vi "LoadUtilization.vi"(0 "base path":path=path "c:/temp", 2 "machine":string="QAMT01") -> (7 "appended array":string[](array[string]), 9 "error out":errorcluster)   [LabVIEW 2012]
uses:
  <vilib>/addons/database/Connection.llb/DB Tools Open Connec (Path).vi
  <vilib>/Utility/file.llb/Read From Spreadsheet File (string).vi
  <vilib>/addons/database/Connection.llb/Conn Execute.vi
  <vilib>/addons/database/Recordset.llb/Rec Fetch Integer Data (R).vi
  <vilib>/addons/database/Recordset.llb/Rec Destroy - Connection.vi
  <vilib>/regexp/Match Regular Expression.xnode
  <vilib>/addons/database/NI_Database_API.lvlib
panel:
  out "error out 4":errorcluster
  out "error out 3":errorcluster
  out "input cluster 2":T1
  out "error out 2":errorcluster
  out "trimmed string":string
  out "output cluster":T1
  out "data":i32
  out "concatenated string":string
  out "x = y?":bool
  in  "input cluster":T1
  in  "String":string
  in  "Array":string[](array[string])
  out "filenames":string[](array[string])
  out "Numeric":i32
  in  "date/time string 2":string
  out "all rows":string[][](array[string])
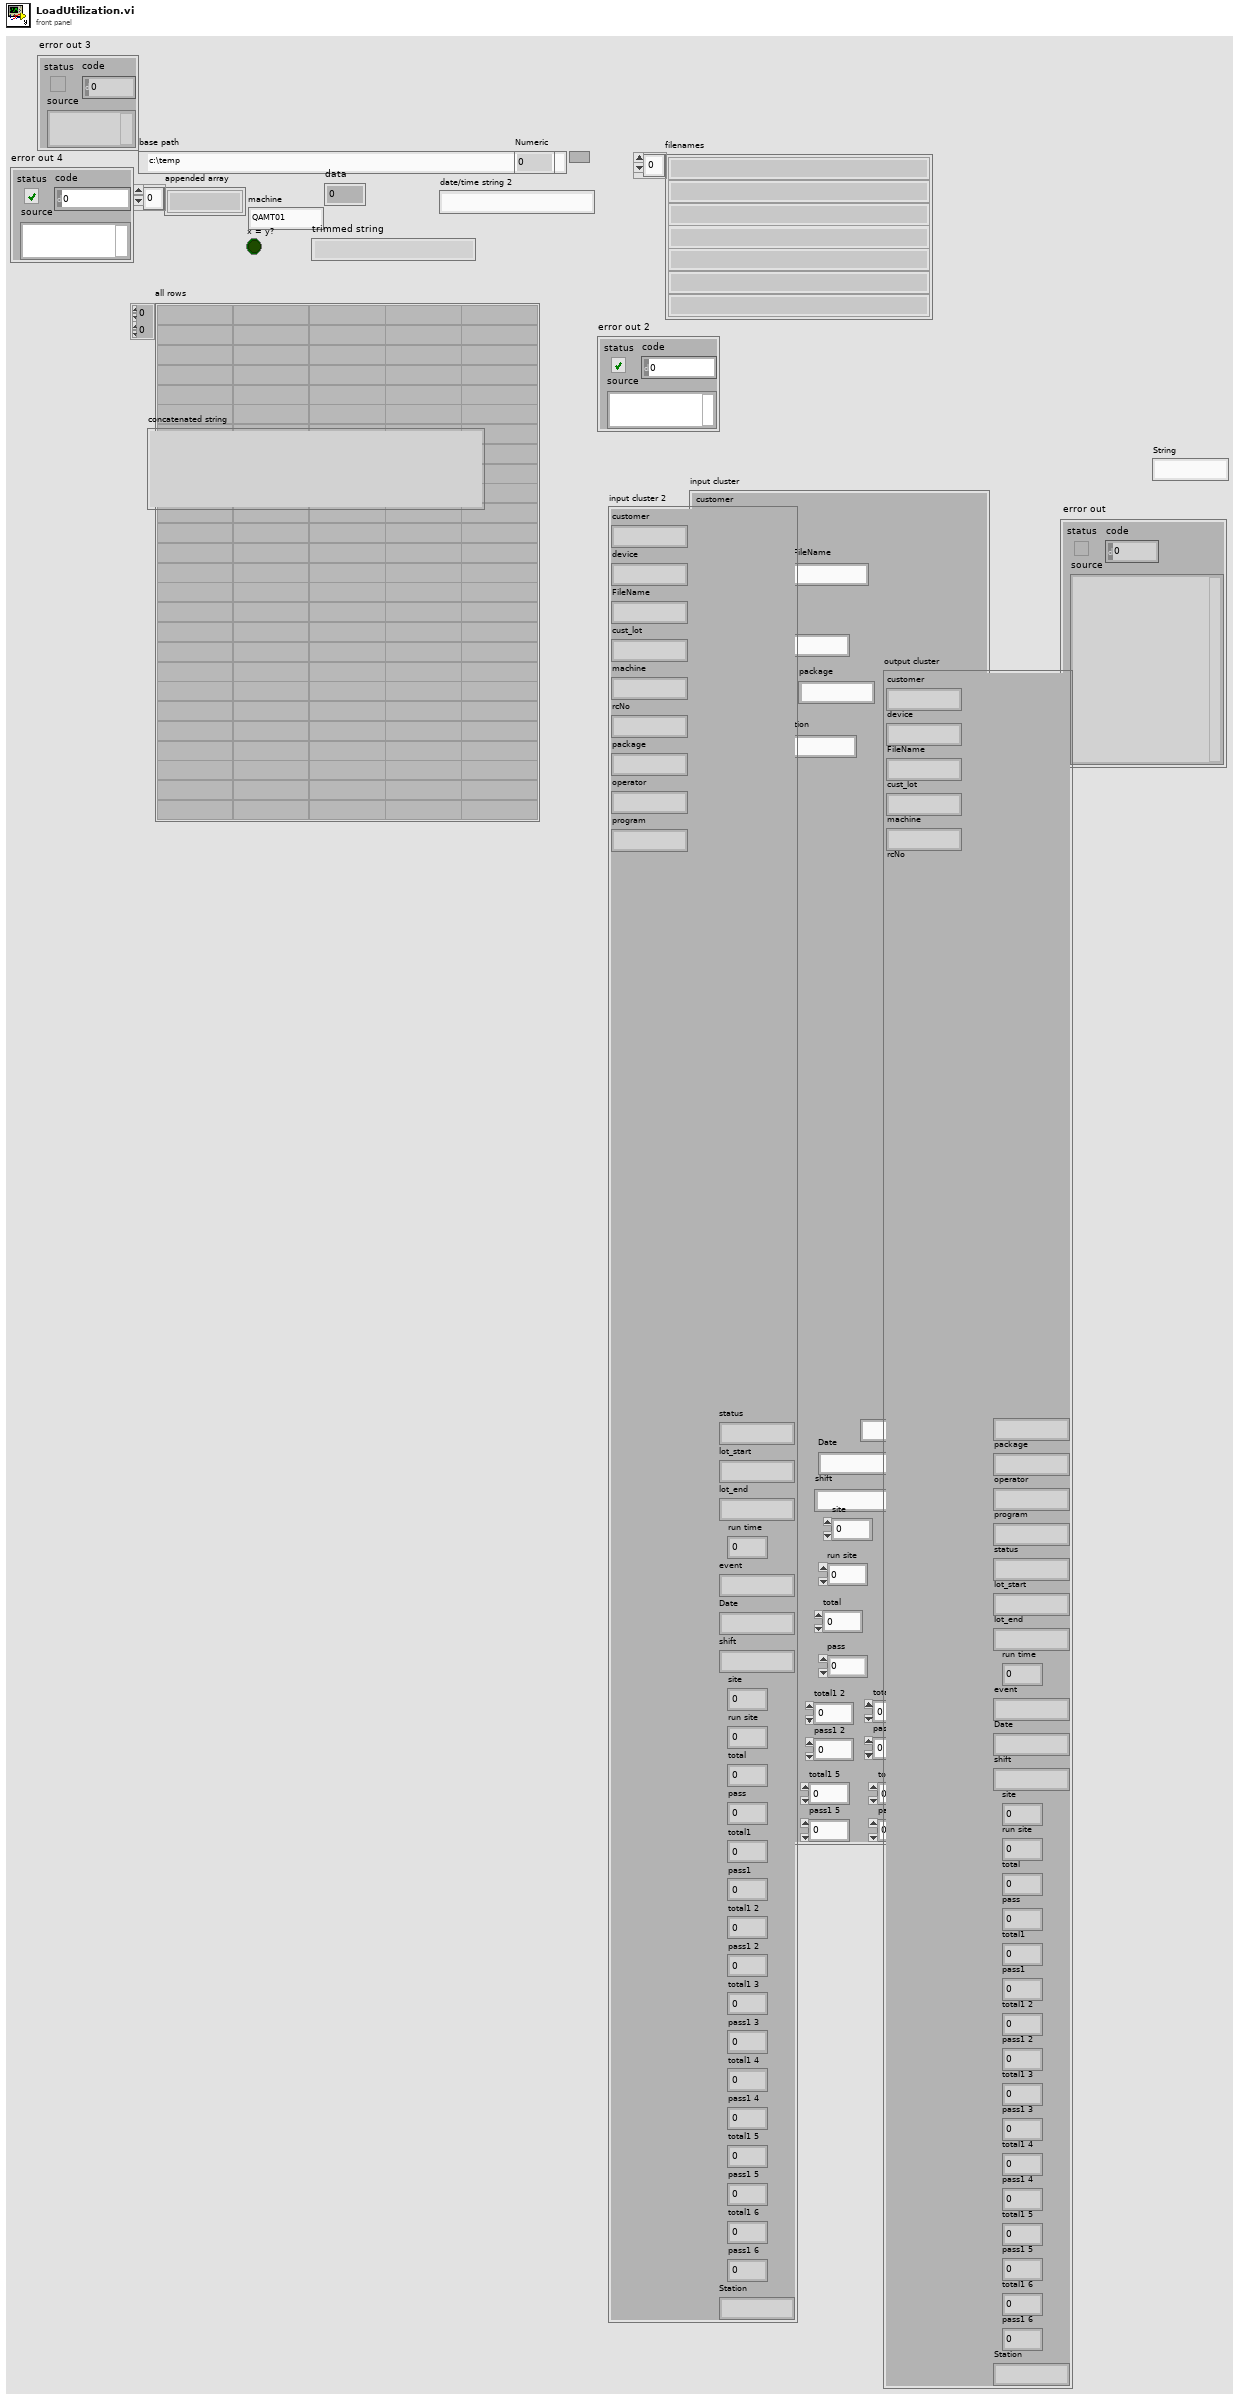
[diagram p1: front panel]
types:
  T1 = cluster{"customer":string, "device":string, "FileName":string, "cust_lot":string, "machine":string, "rcNo":string, "package":string, "operator":string, "program":string, "status":string, "lot_start":string, "lot_end":string, "run time":dbl, "event":string, "Date":string, "shift":string, "site":dbl, "run site ":dbl, "total":dbl, "pass":dbl, "total1":dbl, "pass1":dbl, "total1 2":dbl, "pass1 2":dbl, "total1 3":dbl, "pass1 3":dbl, "total1 4":dbl, "pass1 4":dbl, "total1 5":dbl, "pass1 5":dbl, "total1 6":dbl, "pass1 6":dbl, "Station":string}
  T2 = typedef "NI_Database_API.lvlib/Conn ObjectReference.ctl" = refnum<k1>
  T3 = typedef "NI_Database_API.lvlib/Rec ObjectReference.ctl" = refnum<k1>
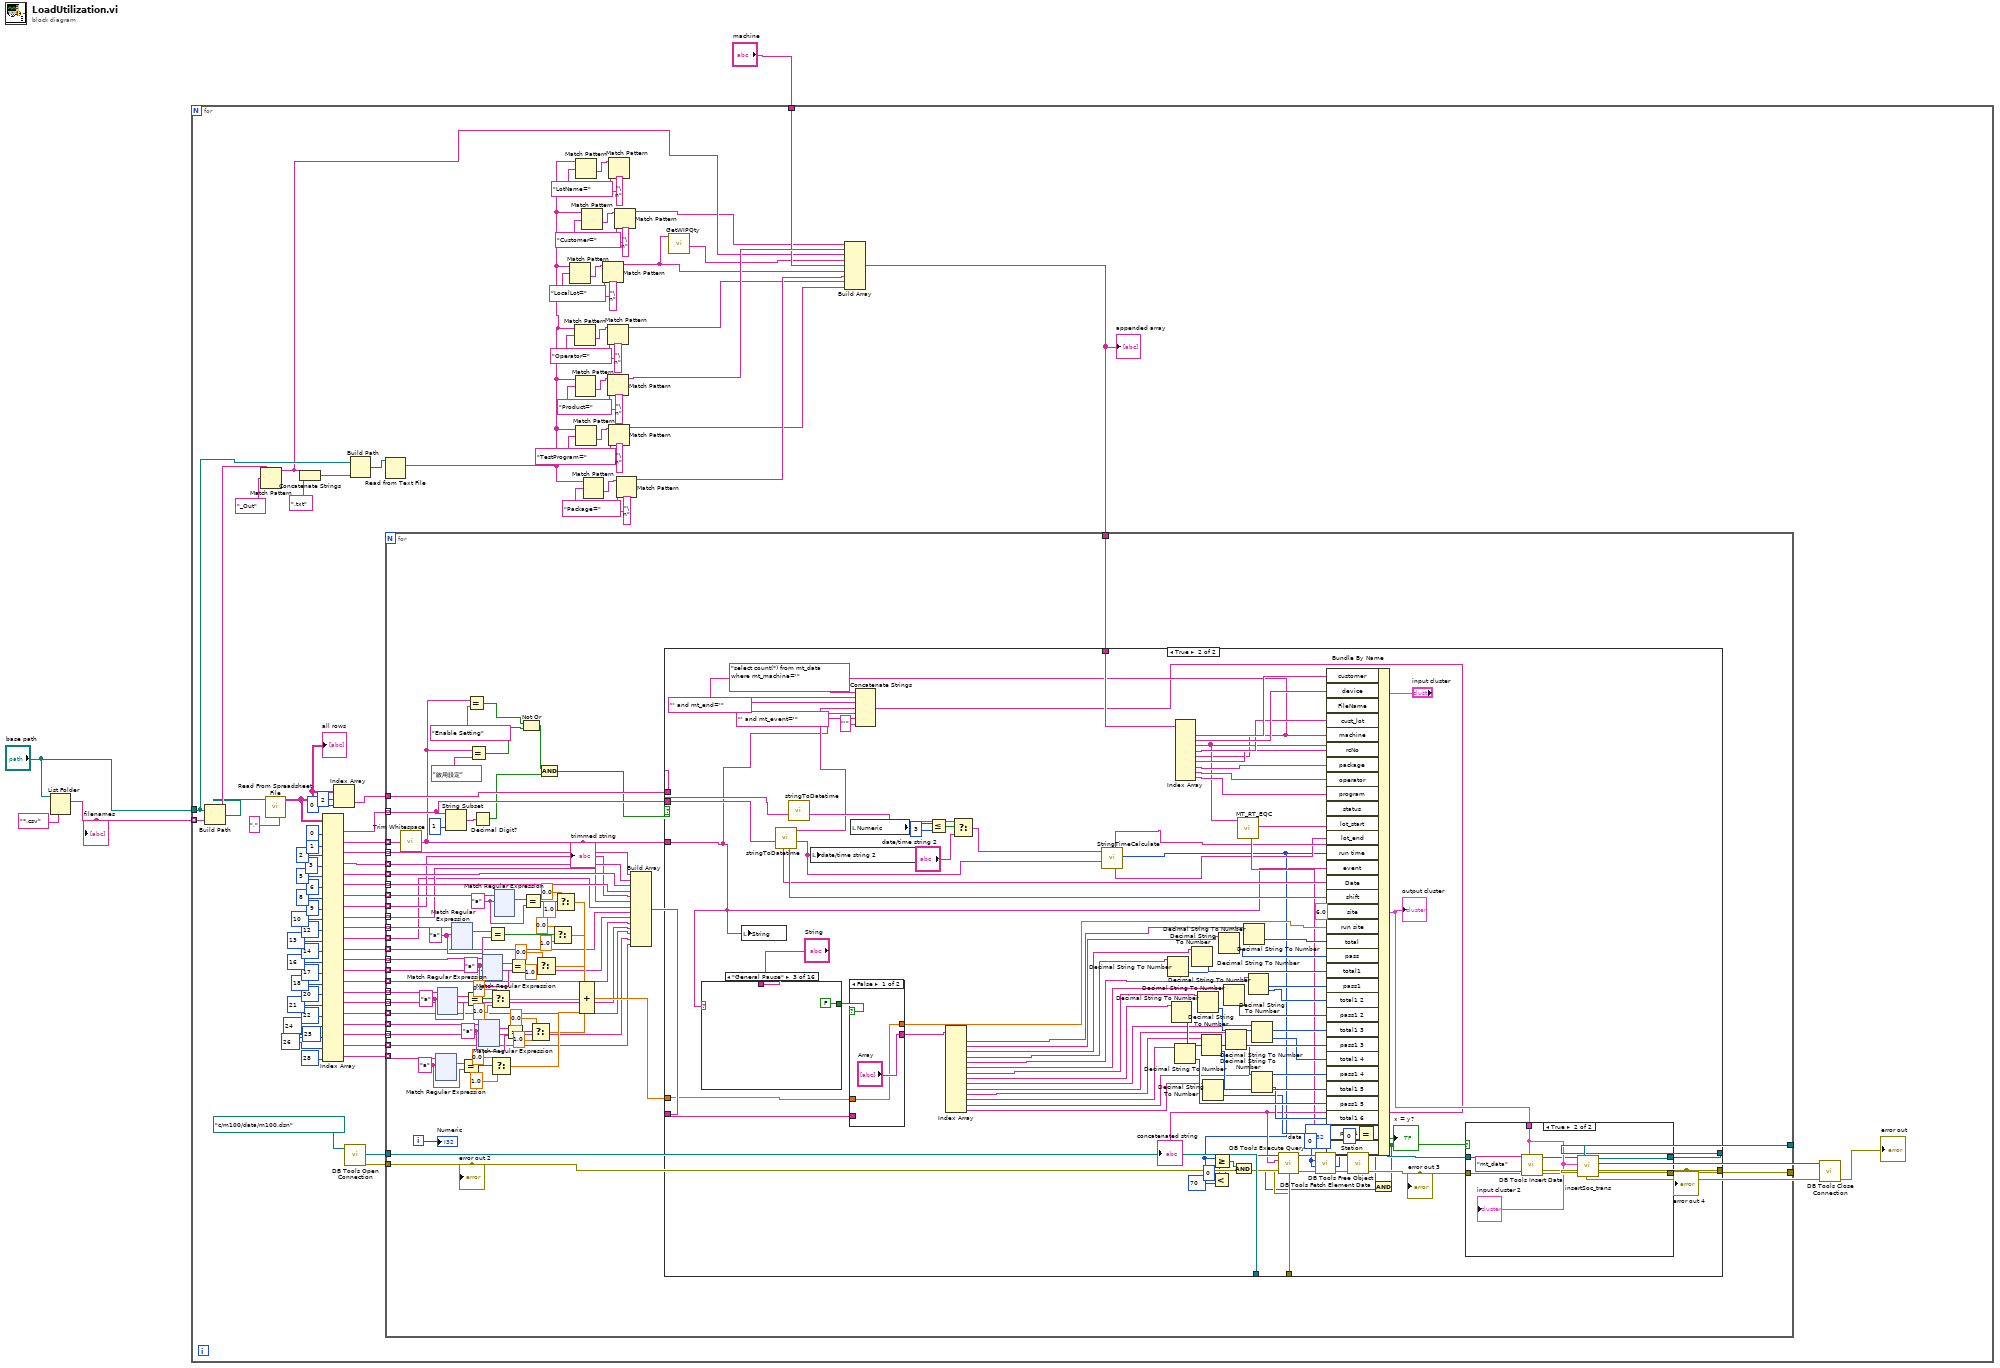
[diagram p0: block diagram]
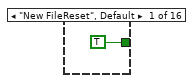
[diagram p5: hidden frame]
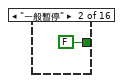
[diagram p6: hidden frame]
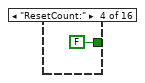
[diagram p7: hidden frame]
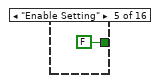
[diagram p8: hidden frame]
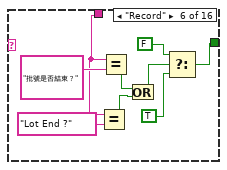
[diagram p9: hidden frame]
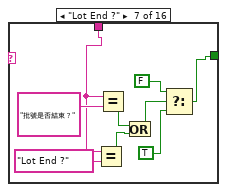
[diagram p10: hidden frame]
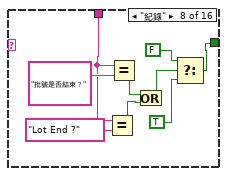
[diagram p11: hidden frame]
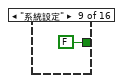
[diagram p12: hidden frame]
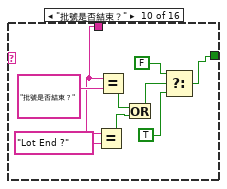
[diagram p13: hidden frame]
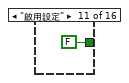
[diagram p14: hidden frame]
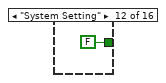
[diagram p15: hidden frame]
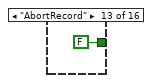
[diagram p16: hidden frame]
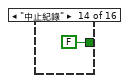
[diagram p17: hidden frame]
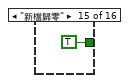
[diagram p18: hidden frame]
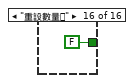
[diagram p19: hidden frame]
diagram:
  n1 = List Folder(path="base path", pattern="*.csv") -> (filenames=w2:string[])  [unwired: 2 in, 3 out]
  "filenames" <- w2
  n2 = for {
    tunnel: "base path" -> [w16]
    tunnel: w2 -> [w48] mode=indexing
    tunnel: "machine" -> [w9]
    n3 = Build Path(base path=w16, name or relative path=w48) -> (appended path=w46:path)
    n4 = Match Pattern(string=w48, regular expression="_Out") -> (before substring=w6:string)  [unwired: 1 in, 3 out]
    n5 = call-poly <vilib>:"Read From Spreadsheet File.vi"("delimiter (\\t)"="," ("delimiter (\\t)"), "file path (dialog if empty)"=w46) -> ("all rows"=w86:string[][])  [unwired: 5 in, 4 out]
    "all rows" <- w86
    n6 = Concatenate Strings(w6, ".txt" ("string")) -> (w45:string)
    n7 = Index Array(array=w86, index (col) #1=0 ("disabled index (col)"), index (col) #2=1 ("index (col)"), index (col) #3=2 ("index (col)"), index (col) #4=3 ("index (col)"), index (col) #5=5 ("index (col)"), index (col) #6=6 ("index (col)"), index (col) #7=8 ("index (col)"), index (col) #8=9 ("index (col)"), index (col) #9=10 ("index (col)"), index (col) #10=12 ("index (col)"), index (col) #11=13 ("index (col)"), index (col) #12=14 ("index (col)"), index (col) #13=16 ("index (col)"), index (col) #14=17 ("index (col)"), index (col) #15=18 ("index (col)"), index (col) #16=20 ("index (col)"), index (col) #17=21 ("index (col)"), index (col) #18=22 ("index (col)"), index (col) #19=24 ("index (col)"), index (col) #20=25 ("index (col)"), index (col) #21=26 ("index (col)"), index (col) #22=28 ("index (col)")) -> (element #1=w90:string[], element #2=w89:string[], element #3=w88:string[], element #4=w87:string[], element #5=w69:string[], element #6=w68:string[], element #7=w61:string[], element #8=w59:string[], element #9=w58:string[], element #10=w62:string[], element #11=w57:string[], element #12=w56:string[], element #13=w60:string[], element #14=w55:string[], element #15=w54:string[], element #16=w63:string[], element #17=w53:string[], element #18=w52:string[], element #19=w64:string[], element #20=w51:string[], element #21=w50:string[], element #22=w65:string[])  [unwired: 22 in]
    n8 = Index Array(array=w86, index (row)=2, index (col)=0 ("disabled index (col)")) -> (element=w83:string)
    n9 = call-poly <vilib>:"DB Tools Open Connection.vi"("connection information"=path "c:/m100/data/m100.dsn") -> ("error out"=w13:errorcluster, "connection reference"=w14:T2)  [unwired: 7 in]
    n10 = Build Path(base path=w16, name or relative path=w45) -> (appended path=w17:path)
    n11 = Read from Text File(file (use dialog)=w17) -> (text=w23:string)  [unwired: 3 in, 3 out]
    n12 = Match Pattern(string=w23, regular expression="LocalLot=") -> (after substring=w37:string)  [unwired: 1 in, 3 out]
    n13 = Match Pattern(string=w23, regular expression="Operator=") -> (after substring=w34:string)  [unwired: 1 in, 3 out]
    n14 = Match Pattern(string=w23, regular expression="Product=") -> (after substring=w31:string)  [unwired: 1 in, 3 out]
    n15 = Match Pattern(string=w23, regular expression="LotName=") -> (after substring=w43:string)  [unwired: 1 in, 3 out]
    n16 = Match Pattern(string=w23, regular expression="TestProgram=") -> (after substring=w28:string)  [unwired: 1 in, 3 out]
    n17 = Match Pattern(string=w23, regular expression="Customer=") -> (after substring=w40:string)  [unwired: 1 in, 3 out]
    n18 = Match Pattern(string=w23, regular expression="Package=") -> (after substring=w25:string)  [unwired: 1 in, 3 out]
    n19 = Match Pattern(string=w37, regular expression="\n") -> (before substring=w7:string)  [unwired: 1 in, 3 out]
    n20 = Match Pattern(string=w34, regular expression="\n") -> (before substring=w18:string)  [unwired: 1 in, 3 out]
    n21 = Match Pattern(string=w31, regular expression="\n") -> (before substring=w20:string)  [unwired: 1 in, 3 out]
    n22 = Match Pattern(string=w43, regular expression="\n") -> ()  [unwired: 1 in, 4 out]
    n23 = Match Pattern(string=w28, regular expression="\n") -> (before substring=w19:string)  [unwired: 1 in, 3 out]
    n24 = Match Pattern(string=w40, regular expression="\n") -> (before substring=w5:string)  [unwired: 1 in, 3 out]
    n25 = Match Pattern(string=w25, regular expression="\n") -> (before substring=w22:string)  [unwired: 1 in, 3 out]
    n26 = call "GetWIPQty.vi"("Lotno"=w7) -> ("lotno"=w8:string)  [unwired: 2 in, 8 out]
    n27 = Build Array(w5, w20, w6, w8, w9, w7, w22, w18, w19) -> (w21:string[])
    "appended array" <- w21
    n28 = for {
      tunnel: w90 -> [w173] mode=indexing
      tunnel: w89 -> [w106] mode=indexing
      tunnel: w88 -> [w127] mode=indexing
      tunnel: w87 -> [w126] mode=indexing
      tunnel: w83 -> [w172]
      tunnel: w69 -> [w125] mode=indexing
      tunnel: w68 -> [w124] mode=indexing
      tunnel: w65 -> [w170] mode=indexing
      tunnel: w64 -> [w165] mode=indexing
      tunnel: w63 -> [w166] mode=indexing
      tunnel: w62 -> [w168] mode=indexing
      tunnel: w61 -> [w169] mode=indexing
      tunnel: w60 -> [w167] mode=indexing
      tunnel: w59 -> [w123] mode=indexing
      tunnel: w58 -> [w122] mode=indexing
      tunnel: w57 -> [w121] mode=indexing
      tunnel: w56 -> [w120] mode=indexing
      tunnel: w55 -> [w119] mode=indexing
      tunnel: w54 -> [w118] mode=indexing
      tunnel: w53 -> [w117] mode=indexing
      tunnel: w52 -> [w116] mode=indexing
      tunnel: w51 -> [w115] mode=indexing
      tunnel: w50 -> [w114] mode=indexing
      tunnel: w21 -> [w112]
      tunnel: w14 -> [w111]
      tunnel: w13 -> [w110]
      tunnel: [w109] -> w12
      tunnel: [w108] -> w11
      i -> [w171]
      w161 = "a" ("regular expression")
      w159 = "a" ("regular expression")
      w154 = "a" ("regular expression")
      w157 = "a" ("regular expression")
      w128 = "a" ("regular expression")
      w156 = "a" ("regular expression")
      n29 = call <vilib>:"Trim Whitespace.vi"("string"=w106) -> ("trimmed string"=w105:string)  [unwired: 1 in]
      "trimmed string" <- w105
      n30 = xnode "Match Regular Expression"("input string"=w170, "regular expression"=w161) -> ("whole match"=w162:string)  [unwired: 4 in, 4 out]
      n31 = xnode "Match Regular Expression"("input string"=w166, "regular expression"=w154) -> ("whole match"=w155:string)  [unwired: 4 in, 4 out]
      n32 = String Subset(string=w173, length (rest)=1 ("length (rest)")) -> (substring=w174:string)  [unwired: 1 in]
      n33 = xnode "Match Regular Expression"("input string"=w168, "regular expression"=w128) -> ("whole match"=w163:string)  [unwired: 4 in, 4 out]
      n34 = Equal?(x=w162, y=w161) -> (x = y?=w148:bool)
      n35 = Equal?(x=w155, y=w154) -> (x = y?=w150:bool)
      n36 = Equal?(x=w105, y="Enable Setting") -> (x = y?=w103:bool)
      n37 = Equal?(x=w105, y="啟用設定") -> (x = y?=w102:bool)
      n38 = Decimal Digit?(1:w174) -> (0:w100:bool)
      n39 = xnode "Match Regular Expression"("input string"=w165, "regular expression"=w159) -> ("whole match"=w160:string)  [unwired: 4 in, 4 out]
      n40 = xnode "Match Regular Expression"("input string"=w167, "regular expression"=w157) -> ("whole match"=w158:string)  [unwired: 4 in, 4 out]
      n41 = Equal?(x=w163, y=w128) -> (x = y?=w152:bool)
      n42 = Select(t=0.0, s=w150, f=1.0) -> (s? t:f=w132:dbl)
      n43 = Select(t=0.0, s=w148, f=1.0) -> (s? t:f=w131:dbl)
      n44 = xnode "Match Regular Expression"("input string"=w169, "regular expression"=w156) -> ("whole match"=w164:string)  [unwired: 4 in, 4 out]
      n45 = Equal?(x=w160, y=w159) -> (x = y?=w149:bool)
      n46 = Equal?(x=w158, y=w157) -> (x = y?=w151:bool)
      n47 = Not Or(1:w102, 2:w103) -> (0:w101:bool)
      n48 = Equal?(x=w164, y=w156) -> (x = y?=w153:bool)
      n49 = Select(t=0.0, s=w149, f=1.0) -> (s? t:f=w130:dbl)
      n50 = Select(t=0.0, s=w151, f=1.0) -> (s? t:f=w133:dbl)
      n51 = And(x=w101, y=w100) -> (x .and. y?=w99:bool)
      n52 = Select(t=0.0, s=w152, f=1.0) -> (s? t:f=w134:dbl)
      n53 = Select(t=0.0, s=w153, f=1.0) -> (s? t:f=w135:dbl)
      n54 = Compound Arithmetic op=ADD(w135, w134, w133, w132, w130, w131) -> (w129:dbl)
      n55 = Build Array(w127, w126, w125, w124, w123, w122, w121, w120, w119, w118, w117, w116, w115, w114) -> (w113:string[])
      n56 = case shown="True" w99 {
        tunnel: w173 -> [_ w848]
        tunnel: w105 -> [_ w844]
        tunnel: w172 -> [_ w929]
        tunnel: w129 -> [_ w927]
        tunnel: w113 -> [_ w926]
        tunnel: w112 -> [_ w893]
        tunnel: w111 -> [w843 w875]
        tunnel: w110 -> [w842 w876]
        tunnel: [w843 w865] -> w109
        tunnel: [w842 w883] -> w108
        frame False {
        }
        frame True {
          w866 = 0
          n57 = case shown="\"General Pause\"" w844 {
            tunnel: [TRUE FALSE ("t") FALSE ("t") FALSE FALSE w953 w962 w974 FALSE w981 FALSE ("t") FALSE ("t") FALSE ("t") FALSE ("t") TRUE FALSE] -> w928
            tunnel: "String" -> [_ _ _ _ _ w954 w963 w971 _ w982 _ _ _ _ _ _]
            frame "New FileReset", Default {
            }
            frame "一般暫停" {
            }
            frame "General Pause" {
            }
            frame "ResetCount:" {
            }
            frame "Enable Setting" {
            }
            frame "Record" {
              n58 = Equal?(x=w954, y="Lot End ?") -> (x = y?=w958:bool)
              n59 = Equal?(x=w954, y="批號是否結束？") -> (x = y?=w959:bool)
              n60 = Or(x=w959, y=w958) -> (x .or. y?=w957:bool)
              n61 = Select(t=FALSE, s=w957, f=TRUE) -> (s? t:f=w953:bool)
            }
            frame "Lot End ?" {
              n62 = Equal?(x=w963, y="Lot End ?") -> (x = y?=w967:bool)
              n63 = Equal?(x=w963, y="批號是否結束？") -> (x = y?=w968:bool)
              n64 = Or(x=w968, y=w967) -> (x .or. y?=w966:bool)
              n65 = Select(t=FALSE, s=w966, f=TRUE) -> (s? t:f=w962:bool)
            }
            frame "紀錄" {
              n66 = Equal?(x=w971, y="Lot End ?") -> (x = y?=w976:bool)
              n67 = Equal?(x=w971, y="批號是否結束？") -> (x = y?=w977:bool)
              n68 = Or(x=w977, y=w976) -> (x .or. y?=w975:bool)
              n69 = Select(t=FALSE, s=w975, f=TRUE) -> (s? t:f=w974:bool)
            }
            frame "系統設定" {
            }
            frame "批號是否結束？" {
              n70 = Equal?(x=w982, y="Lot End ?") -> (x = y?=w986:bool)
              n71 = Equal?(x=w982, y="批號是否結束？") -> (x = y?=w987:bool)
              n72 = Or(x=w987, y=w986) -> (x .or. y?=w985:bool)
              n73 = Select(t=FALSE, s=w985, f=TRUE) -> (s? t:f=w981:bool)
            }
            frame "啟用設定" {
            }
            frame "System Setting" {
            }
            frame "AbortRecord" {
            }
            frame "中止紀錄" {
            }
            frame "新檔歸零" {
            }
            frame "重設數量︰" {
            }
          }
          n74 = local write "String"(w844) -> ()
          n75 = call "stringToDatetime.vi"("input string"=w848) -> ("date/time string"=w859:string, "sqltime string"=w849:string, "Shift"=w862:string, "ShiftDate"=w861:string)  [unwired: 7 in]
          n76 = call "stringToDatetime.vi"("input string"=w929) -> ("date/time string"=w930:string)  [unwired: 7 in, 3 out]
          n77 = local write "date/time string 2"(w859) -> ()
          n78 = case shown="False" w928 {
            tunnel: [w944 w947] -> w896
            tunnel: w927 -> [w944 w947]
            tunnel: ["Array" w946] -> w925
            tunnel: w926 -> [_ w946]
            frame False {
            }
            frame True {
            }
          }
          n79 = local read "Numeric"() -> (w933:i32)
          n80 = Less Or Equal?(x=w933, y=3) -> (x <= y?=w931:bool)
          n81 = Index Array(array=w925) -> (element #1=w897:string, element #2=w898:string, element #3=w899:string, element #4=w900:string, element #5=w902:string, element #6=w903:string, element #7=w904:string, element #8=w905:string, element #9=w906:string, element #10=w907:string, element #11=w908:string, element #12=w909:string, element #13=w901:string, element #14=w910:string)  [unwired: 14 in]
          n82 = Select(t=w930, s=w931, f="date/time string 2") -> (s? t:f=w881:string)
          n83 = call "StringTimeCalculate.vi"("End Date"=w859, "Start Date"=w881) -> ("Minutes"=w847:i32, "SQLEndTime"=w850:string, "SQLStartTime"=w851:string)  [unwired: 7 in]
          n84 = Decimal String To Number(string=w900) -> (number=w921:i32)  [unwired: 2 in, 1 out]
          n85 = Decimal String To Number(string=w905) -> (number=w917:i32)  [unwired: 2 in, 1 out]
          n86 = Decimal String To Number(string=w909) -> (number=w913:i32)  [unwired: 2 in, 1 out]
          n87 = Index Array(array=w893) -> (element #1=w892:string, element #2=w891:string, element #3=w884:string, element #4=w890:string, element #5=w871:string, element #6=w889:string, element #7=w888:string, element #8=w887:string, element #9=w886:string)  [unwired: 9 in]
          n88 = Concatenate Strings("select count(*) from mt_data where mt_machine='" ("string"), w871, "' and mt_end='" ("string"), w849, "' and mt_event='" ("string"), w844, "'" ("string")) -> (w867:string)
          "concatenated string" <- w867
          n89 = Decimal String To Number(string=w899) -> (number=w922:i32)  [unwired: 2 in, 1 out]
          n90 = Decimal String To Number(string=w904) -> (number=w918:i32)  [unwired: 2 in, 1 out]
          n91 = Decimal String To Number(string=w908) -> (number=w914:i32)  [unwired: 2 in, 1 out]
          n92 = Decimal String To Number(string=w910) -> (number=w911:i32)  [unwired: 2 in, 1 out]
          n93 = Less?(x=w847, y=70) -> (x < y?=w855:bool)
          n94 = Greater Or Equal?(x=w847, y=0) -> (x >= y?=w856:bool)
          n95 = Decimal String To Number(string=w898) -> (number=w923:i32)  [unwired: 2 in, 1 out]
          n96 = Decimal String To Number(string=w903) -> (number=w919:i32)  [unwired: 2 in, 1 out]
          n97 = Decimal String To Number(string=w907) -> (number=w915:i32)  [unwired: 2 in, 1 out]
          n98 = And(x=w856, y=w855) -> (x .and. y?=w852:bool)
          n99 = call "MT_RT_EQC.vi"("input string"=w884) -> ("Station"=w885:string, "STN"=w860:string)  [unwired: 6 in, 3 out]
          n100 = Decimal String To Number(string=w897) -> (number=w924:i32)  [unwired: 2 in, 1 out]
          n101 = Decimal String To Number(string=w902) -> (number=w920:i32)  [unwired: 2 in, 1 out]
          n102 = Decimal String To Number(string=w906) -> (number=w916:i32)  [unwired: 2 in, 1 out]
          n103 = Decimal String To Number(string=w901) -> (number=w912:i32)  [unwired: 2 in, 1 out]
          n104 = call-poly <vilib>:"DB Tools Execute Query.vi"("error in (no error)"=w876, "SQL query"=w867, "connection reference"=w875) -> ("error out"=w880:errorcluster, "recordset reference"=w879:T3)  [unwired: 5 in]
          n105 = call-poly <vilib>:"DB Tools Fetch Element Data.vi"("error in (no error)"=w880, "type"=w866, "column index"=w866, "recordset reference"=w879) -> ("error out"=w878:errorcluster, "data"=w864:i32, "recordset reference out"=w877:T3)  [unwired: 3 in]
          "data" <- w864
          n106 = Bundle By Name(cluster="input cluster", "customer"=w892, "device"=w891, "FileName"=w884, "cust_lot"=w890, "machine"=w871, "rcNo"=w889, "package"=w888, "operator"=w887, "program"=w886, "status"=w885, "lot_start"=w851, "lot_end"=w850, "run time"=w847, "event"=w844, "Date"=w861, "shift"=w862, "site"=6.0, "run site"=w896, "total"=w924, "pass"=w923, "total1"=w922, "pass1"=w921, "total1 2"=w920, "pass1 2"=w919, "total1 3"=w918, "pass1 3"=w917, "total1 4"=w916, "pass1 4"=w915, "total1 5"=w914, "pass1 5"=w913, "total1 6"=w912, "pass1 6"=w911, "Station"=w860) -> (w882:T1)
          "output cluster" <- w882
          n107 = call-poly <vilib>:"DB Tools Free Object.vi"("error in (no error)"=w878, "recordset reference"=w877) -> ("error out"=w873:errorcluster, "connection reference"=w874:T2)  [unwired: 8 in]
          "error out 3" <- w873
          n108 = Equal?(x=w864, y=0) -> (x = y?=w853:bool)
          n109 = And(x=w853, y=w852) -> (x .and. y?=w854:bool)
          "x = y?" <- w854
          n110 = case shown="True" w854 {
            tunnel: w874 -> [w934 w943]
            tunnel: w873 -> [w935 w942]
            tunnel: [w935 w936] -> w883
            tunnel: w882 -> [_ w940]
            tunnel: [w934 w937] -> w865
            frame False {
            }
            frame True {
              n111 = call <vilib>:"DB Tools Insert Data.vi"("data"=w940, "error in (no error)"=w942, "table"="mt_data", "connection reference"=w943) -> ("error out"=w938:errorcluster, "connection reference out"=w939:T2)  [unwired: 6 in]
              n112 = call "insertSoc_trans.vi"("error in (no error)"=w938, "input cluster"=w940, "connection reference"=w939) -> ("error out"=w936:errorcluster, "connection reference out"=w937:T2)  [unwired: 7 in]
              "input cluster 2" <- w940
            }
          }
          "error out 4" <- w883
        }
      }
      "Numeric" <- w171
      "error out 2" <- w110
    }
    n113 = call <vilib>:"DB Tools Close Connection.vi"("error in (no error)"=w11, "connection reference"=w12) -> ("error out"=→"error out":errorcluster)  [unwired: 5 in]
  }
